vi "Get Region.vi"(6 "size":i32=6, 9 "X":i32, 10 "Y":i32, 11 "p[x][y]":i32[][](array[numeric])=[[0, 1, 2, 3, 4, 5], [10, 11, 12, 13, 14, 15], [20, 21, 22, 23, 24, 25], [30, 31, 32, 33, 34, 35], [40, 41, 42, 43, 44, 45], [50, 51, 52, 53, 54, 55]]) -> (4 "Region out[12][12]":i32[][](array[numeric]))   [LabVIEW 2015, in "BTeam.lvclass"]
uses:
  BTeam.lvclass
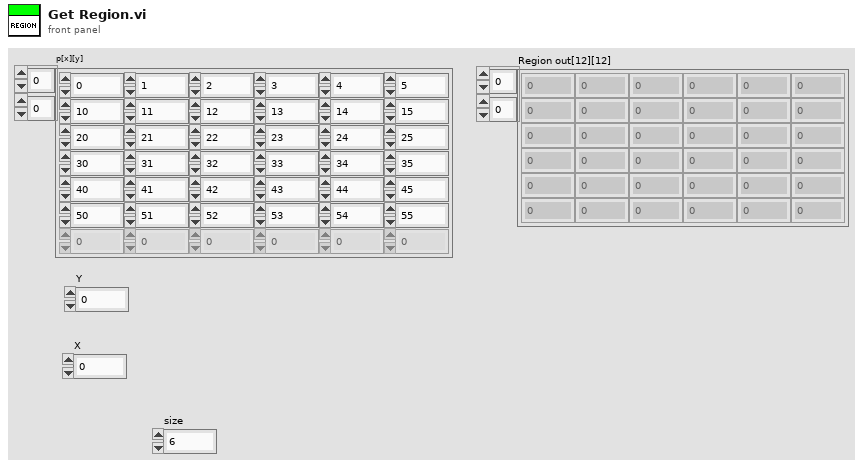
[diagram p1: front panel]
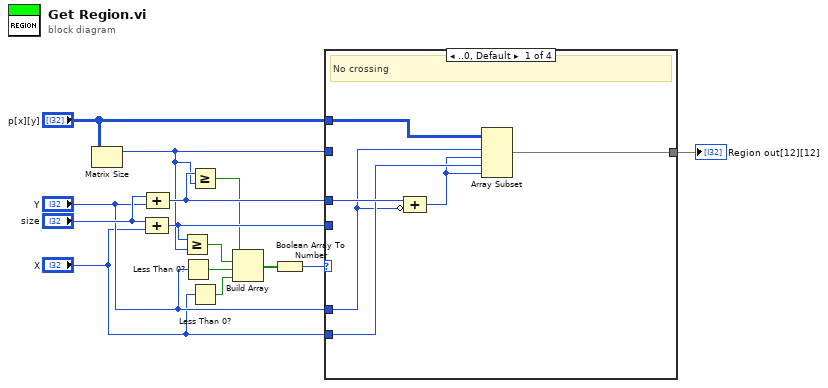
[diagram p0: block diagram]
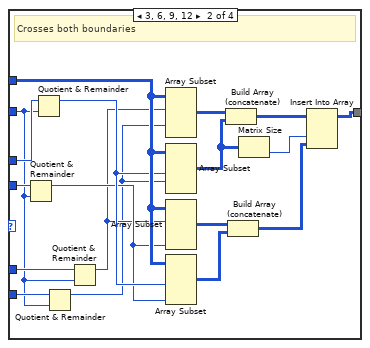
[diagram p2: hidden frame]
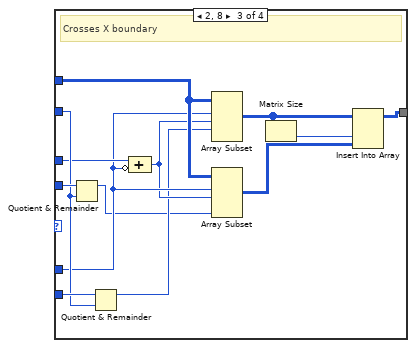
[diagram p3: hidden frame]
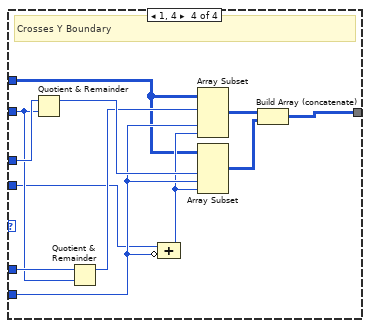
[diagram p4: hidden frame]
diagram:
  n1 = Matrix Size(0:"p[x][y]") -> (1:w3:i32)  [unwired: 1 out]
  n2 = Compound Arithmetic op=ADD("size", "X") -> (w7:i32)
  n3 = Compound Arithmetic op=ADD("size", "Y") -> (w8:i32)
  n4 = Greater Or Equal?(x=w7, y=w3) -> (x >= y?=w4:bool)
  n5 = Less Than 0?(x="Y") -> (x < 0?=w14:bool)
  n6 = Greater Or Equal?(x=w8, y=w3) -> (x >= y?=w5:bool)
  n7 = Less Than 0?(x="X") -> (x < 0?=w13:bool)
  n8 = Build Array(w5, w4, w14, w13) -> (w12:bool[])
  n9 = Boolean Array To Number(Boolean array=w12) -> (number=w11:u32)
  n10 = case shown="..0, Default" w11 {
    tunnel: "p[x][y]" -> [w20 w38 w46 w52]
    tunnel: w8 -> [w18 w28 w45 w61]
    tunnel: [w19 w31 w50 w56] -> w9
    tunnel: w7 -> [_ w36 w51 w54]
    tunnel: "Y" -> [w16 w25 w44 w59]
    tunnel: "X" -> [w17 w23 w49 w55]
    tunnel: w3 -> [_ w22 w48 w57]
    frame ..0, Default {
      # "No crossing"
      n11 = Compound Arithmetic op=ADD(w18, invert w16) -> (w15:i32)
      n12 = Array Subset(array=w20, index (row)=w16, length (row)=w15, index (col)=w17, length (col)=w15) -> (w19:i32[][])
    }
    frame 3, 6, 9, 12 {
      # "Crosses both boundaries"
      n13 = Quotient & Remainder(x=w36, y=w22) -> (x-y*floor(x/y)=w26:i32)  [unwired: 1 out]
      n14 = Quotient & Remainder(x=w28, y=w22) -> (x-y*floor(x/y)=w27:i32)  [unwired: 1 out]
      n15 = Quotient & Remainder(x=w23, y=w22) -> (x-y*floor(x/y)=w21:i32)  [unwired: 1 out]
      n16 = Quotient & Remainder(x=w25, y=w22) -> (x-y*floor(x/y)=w24:i32)  [unwired: 1 out]
      n17 = Array Subset(array=w38, index (row)=w24, index (col)=w21) -> (w37:i32[][])  [unwired: 2 in]
      n18 = Array Subset(array=w38, length (row)=w27, index (col)=w21) -> (w30:i32[][])  [unwired: 2 in]
      n19 = Array Subset(array=w38, index (row)=w24, length (col)=w26) -> (w35:i32[][])  [unwired: 2 in]
      n20 = Array Subset(array=w38, length (row)=w27, length (col)=w26) -> (w34:i32[][])  [unwired: 2 in]
      n21 = Build Array (concatenate)(w37, w30) -> (w33:i32[][])
      n22 = Build Array (concatenate)(w35, w34) -> (w32:i32[][])
      n23 = Matrix Size(0:w30) -> (2:w29:i32)  [unwired: 1 out]
      n24 = Insert Into Array(array=w33, index (col)=w29, new element=w32) -> (w31:i32[][])  [unwired: 1 in]
    }
    frame 2, 8 {
      # "Crosses X boundary"
      n25 = Quotient & Remainder(x=w51, y=w48) -> (x-y*floor(x/y)=w39:i32)  [unwired: 1 out]
      n26 = Quotient & Remainder(x=w49, y=w48) -> (x-y*floor(x/y)=w40:i32)  [unwired: 1 out]
      n27 = Compound Arithmetic op=ADD(w45, invert w44) -> (w43:i32)
      n28 = Array Subset(array=w46, index (row)=w44, length (row)=w43, index (col)=w40) -> (w42:i32[][])  [unwired: 1 in]
      n29 = Array Subset(array=w46, index (row)=w44, length (row)=w43, length (col)=w39) -> (w47:i32[][])  [unwired: 1 in]
      n30 = Matrix Size(0:w42) -> (2:w41:i32)  [unwired: 1 out]
      n31 = Insert Into Array(array=w42, index (col)=w41, new element=w47) -> (w50:i32[][])  [unwired: 1 in]
    }
    frame 1, 4 {
      # "Crosses Y Boundary"
      n32 = Quotient & Remainder(x=w61, y=w57) -> (x-y*floor(x/y)=w60:i32)  [unwired: 1 out]
      n33 = Quotient & Remainder(x=w59, y=w57) -> (x-y*floor(x/y)=w58:i32)  [unwired: 1 out]
      n34 = Compound Arithmetic op=ADD(w54, invert w55) -> (w53:i32)
      n35 = Array Subset(array=w52, index (row)=w58, index (col)=w55, length (col)=w53) -> (w63:i32[][])  [unwired: 1 in]
      n36 = Array Subset(array=w52, length (row)=w60, index (col)=w55, length (col)=w53) -> (w62:i32[][])  [unwired: 1 in]
      n37 = Build Array (concatenate)(w63, w62) -> (w56:i32[][])
    }
  }
  "Region out[12][12]" <- w9
